vi "FSK - Listener.vi"(8 "error in (no error)":errorcluster, 11 "Queues":T1) -> (0 "error out":errorcluster)   [LabVIEW 2013]
uses:
  <vilib>/sound2/lvsound2.llb/Sound Input Task ID.ctl
  <vilib>/sound2/lvsound2.llb/Sound Data Format.ctl
  Object/FSK_OBJ - PROP.ctl
  STYPS/HDR - Queues.ctl
  <vilib>/sound2/lvsound2.llb/Sampling Mode.ctl
  <vilib>/sound2/lvsound2.llb/Sound Input Read (DBL).vi
  <vilib>/Analysis/NI_AALPro.lvlib
panel:
  out "DATA str":string
  out "DATA":string
  out "FSK":T2={"rate (bit/s)"=128.0, "bp (Bit Period)"=1e-06, "f1%"=80.0, "f2%"=20.0, "f1 (1 Freq)"=0.0, "f2 (0 Freq)"=0.0, "t (Time arry)"=[], "y1 (f1 cos arry)"=[], "y2 (f2 cos arry)"=[], "data length (B)"=0, "data size"=0, "sample size"=0.0} {"f2%" format="%#_6f"; "f1%" format="%#_6f"; "sample size" format="%#_13g"; "y2 (f2 cos arry)" format="%#_6f"; "y1 (f1 cos arry)" format="%#_6f"; "t (Time arry)" format="%#_6f"; "f2 (0 Freq)" format="%#_6f"; "f1 (1 Freq)" format="%#_6f"; "bp (Bit Period)" format="%#_13f"; "rate (bit/s)" format="%#_13g"}
  in  "PROPERTIES":T5={"device ID"=0, "number of samples/ch"=2500, "task ID"=0, "sound format"={"sample rate (S/s)"=44100.0, "number of channels"=1, "bits per sample"=16}, "DATA"=[]} {"task ID" format="%.0x"}
  out "i":i32
  out "Waveform":waveform(dbl)[](graph)
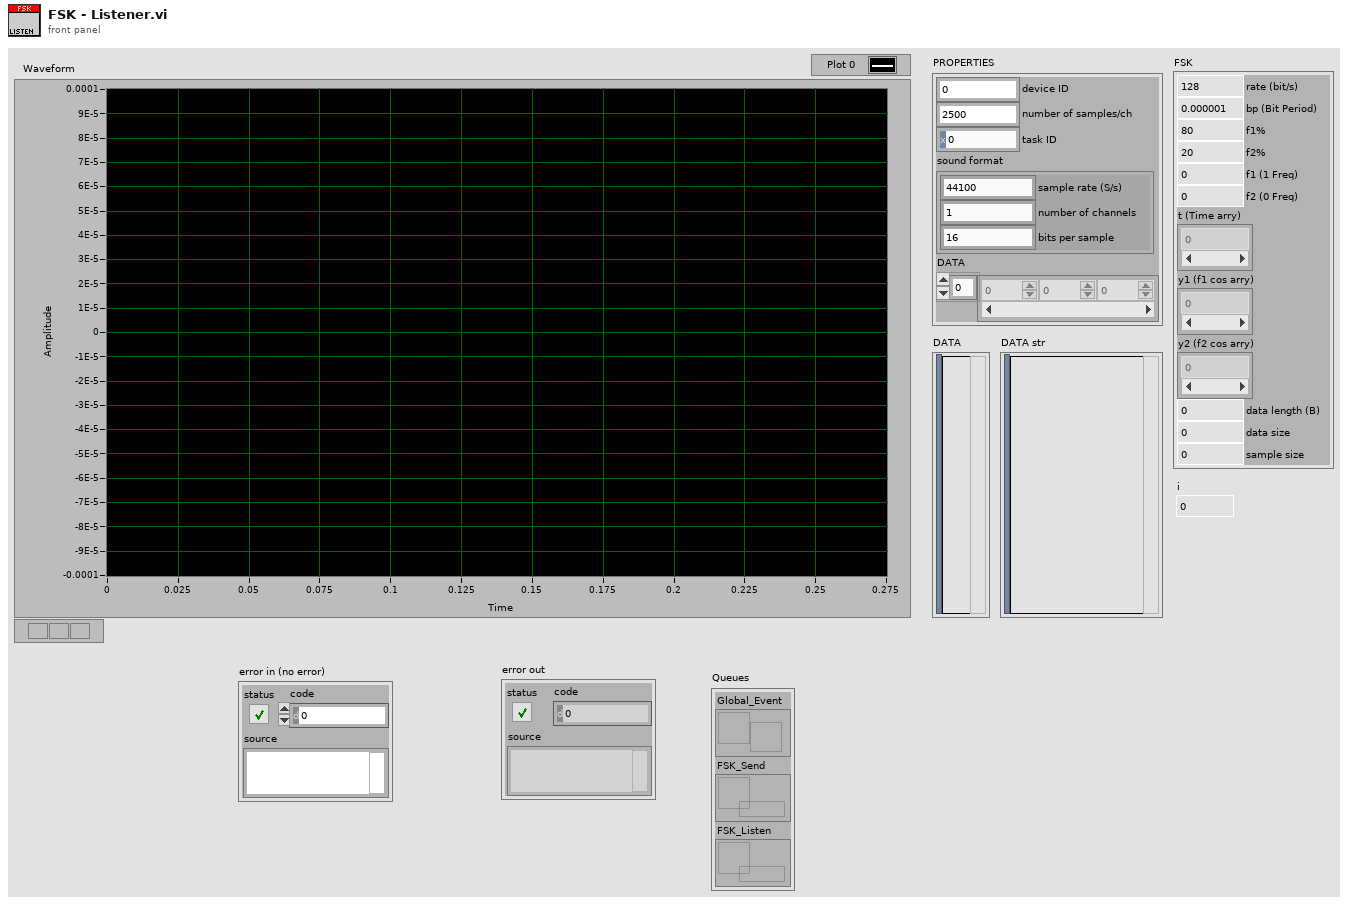
[diagram p1: front panel]
types:
  T1 = typedef "HDR - Queues.ctl" = cluster{"Global_Event":refnum<user-event>, "FSK_Send":refnum<queue>, "FSK_Listen":refnum<queue>}
  T2 = typedef "FSK_OBJ - PROP.ctl" = cluster{"rate (bit/s)":dbl, "bp (Bit Period)":dbl, "f1%":dbl, "f2%":dbl, "f1 (1 Freq)":dbl, "f2 (0 Freq)":dbl, "t (Time arry)":dbl[], "y1 (f1 cos arry)":dbl[], "y2 (f2 cos arry)":dbl[], "data length (B)":i32, "data size":i32, "sample size":dbl}
  T3 = typedef "Sound Input Task ID.ctl" = u32
  T4 = typedef "Sound Data Format.ctl" = cluster{"sample rate (S/s)":dbl, "number of channels":i32, "bits per sample":i32}
  T5 = cluster{"device ID":u32, "number of samples/ch":i32, "task ID":T3, "sound format":T4, "DATA":dbl[]}
  T6 = typedef "Sampling Mode.ctl" = i32
  T7 = typedef "AudioConfig_OBJ - PROP.ctl" = cluster{"Speaker Device ID":u32, "Microphone Device ID":u32, "sound format":T4, "number of samples/ch":i32}
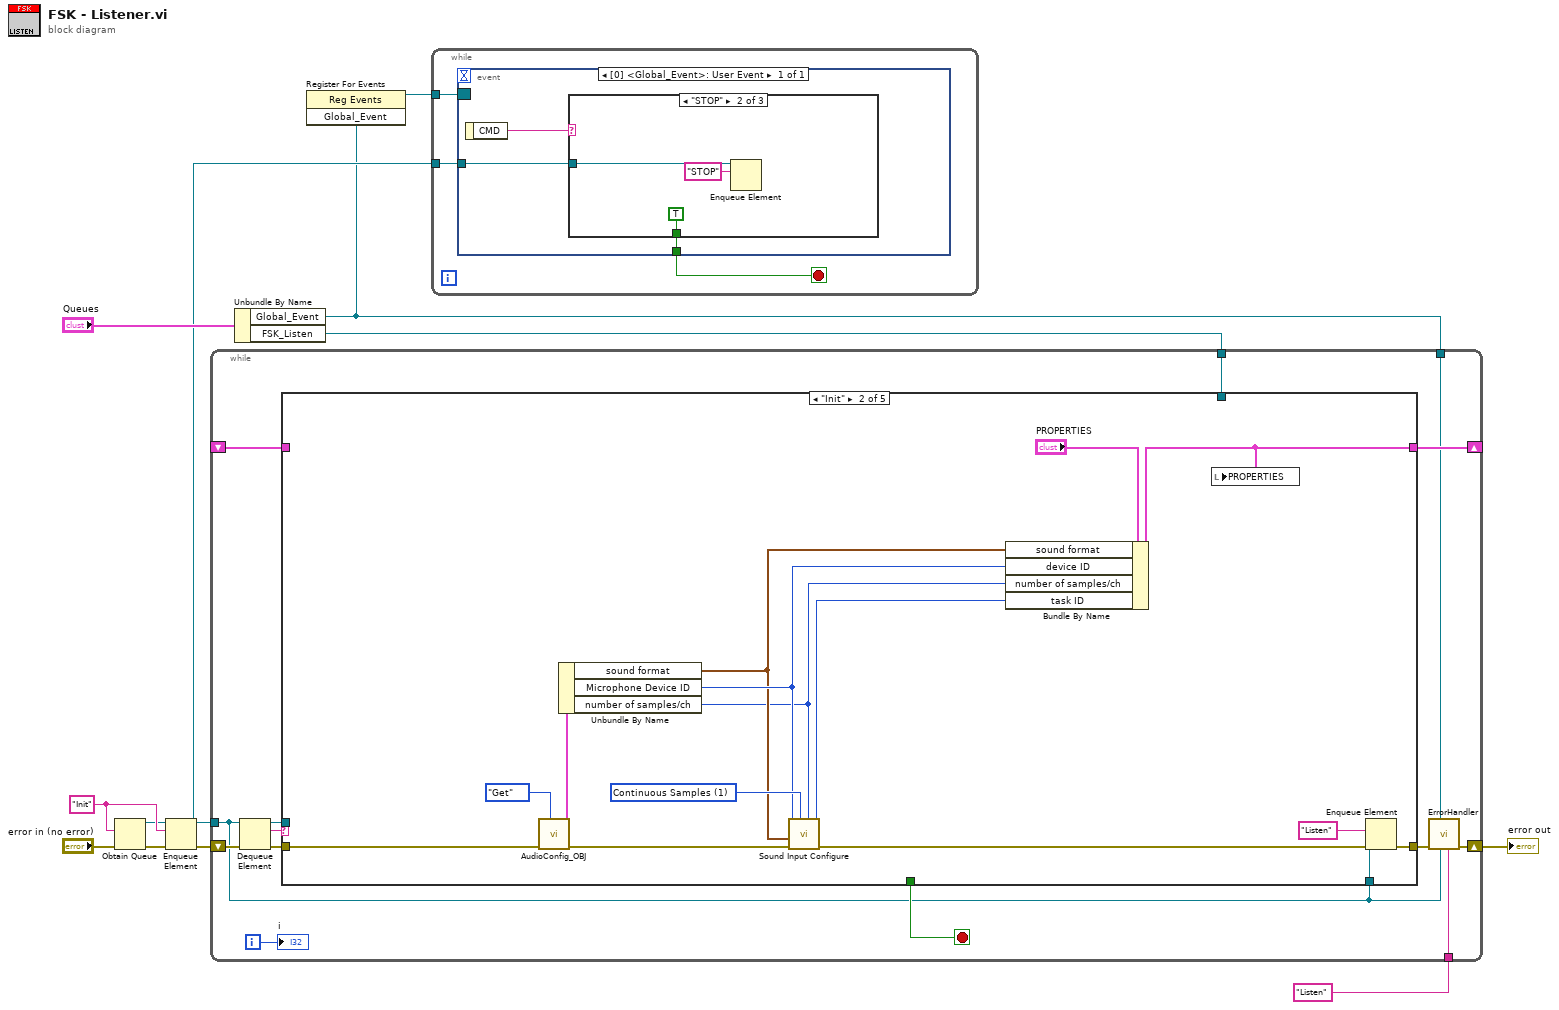
[diagram p0: block diagram]
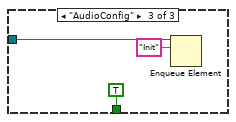
[diagram p3: hidden frame]
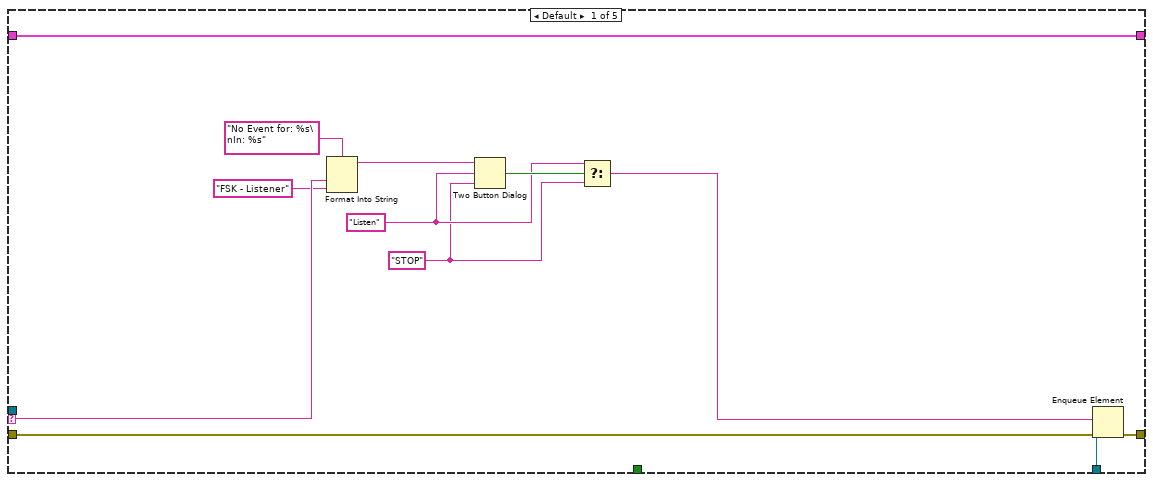
[diagram p4: hidden frame]
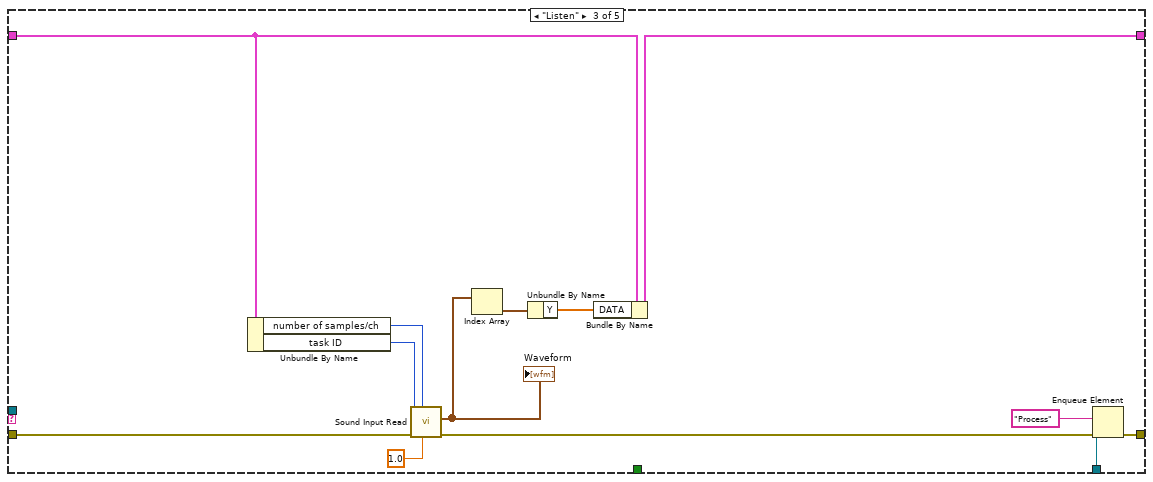
[diagram p5: hidden frame]
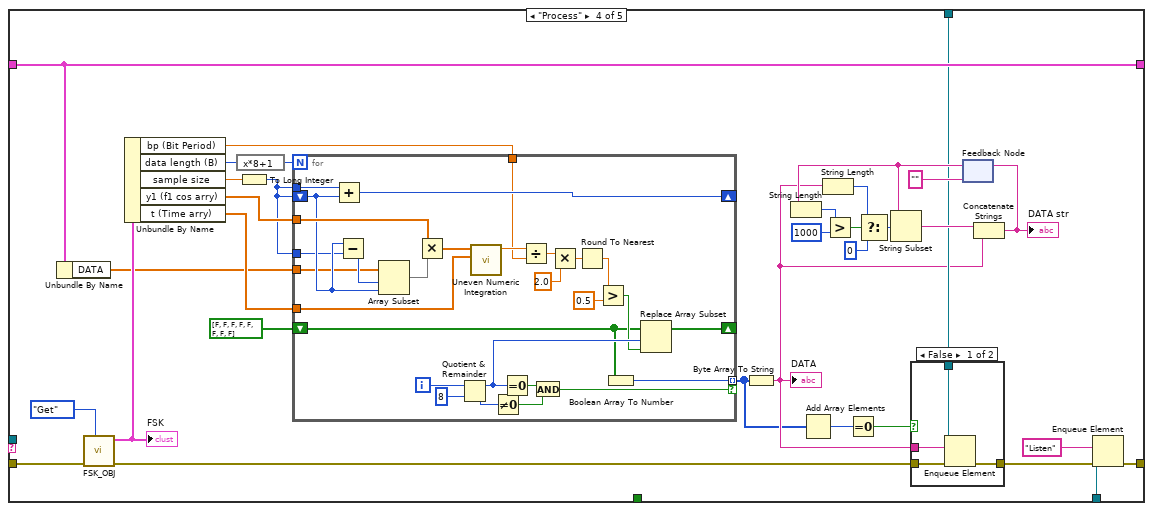
[diagram p6: hidden frame]
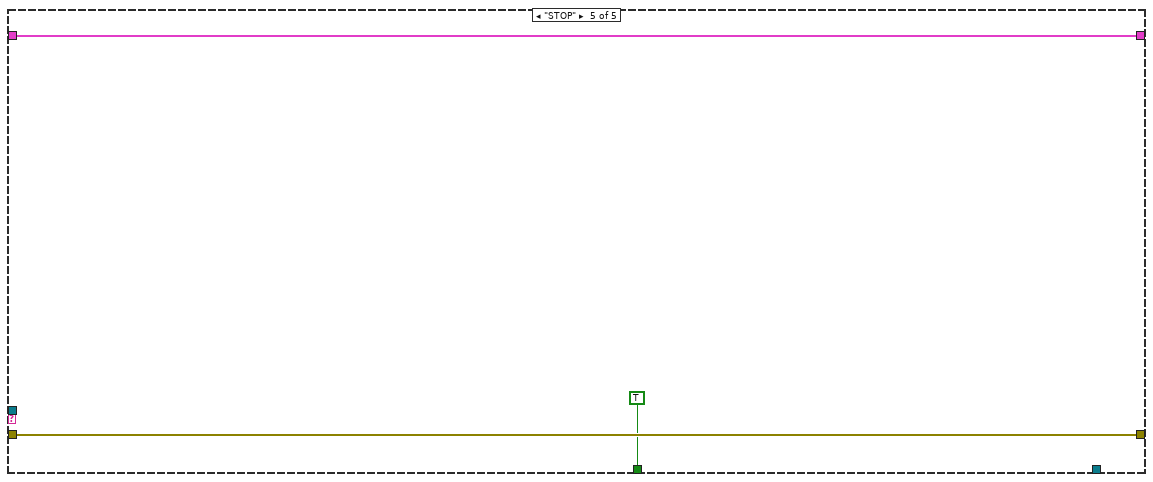
[diagram p8: hidden frame]
diagram:
  w5 = "Init"
  n1 = Obtain Queue(element data type=w5, error in (no error)="error in (no error)") -> (queue out=w4:refnum<queue>, error out=w7:errorcluster)  [unwired: 3 in, 1 out]
  n2 = Enqueue Element(queue=w4, element=w5, error in (no error)=w7) -> (queue out=w3:refnum<queue>, error out=w6:errorcluster)  [unwired: 1 in, 1 out]
  n3 = Unbundle By Name("Queues") -> ("Global_Event"=w2:refnum<user-event>, "FSK_Listen"=w9:refnum<queue>)
  n4 = while {
    shift-right: [w17] -> w12
    shift-left: w6 -> [w22]
    shift-right: [w25] -> _
    shift-left: _ -> [w24]
    tunnel: w9 -> [w23]
    tunnel: w3 -> [w14]
    tunnel: w2 -> [w15]
    tunnel: "Listen" -> [w13]
    i -> [w26]
    stop <- w18 stop-if-true
    n5 = Dequeue Element(queue=w14, error in (no error)=w22) -> (queue out=w20:refnum<queue>, element=w19:string, error out=w21:errorcluster)  [unwired: 1 in, 1 out]
    n6 = case shown="\"Init\"" w19 {
      selector: w19 -> [w37 _ _ _ _]
      tunnel: w21 -> [w29 w49 w66 w98 w134]
      tunnel: [w28 w41 w56 w70 w134] -> w16
      tunnel: [w38 w39 w60 w87 w135] -> w25
      tunnel: w24 -> [w38 _ w64 w87 w135]
      tunnel: w23 -> [_ _ _ w75 _]
      tunnel: w20 -> [_ _ _ _ _]
      tunnel: w14 -> [w30 w43 w55 w68 _]
      tunnel: [_ _ _ _ TRUE] -> w18
      frame Default {
        w32 = "Listen" ("F button name (\"Cancel\")")
        w31 = "STOP" ("F button name (\"Cancel\")")
        n7 = Format Into String(format string="No Event for: %s\nIn: %s", w37, "FSK - Listener" ("input 2")) -> (resulting string=w34:string)  [unwired: 2 in, 1 out]
        n8 = Two Button Dialog(message=w34, 1:w31, 2:w32) -> (T button?=w33:bool)
        n9 = Select(t=w32, s=w33, f=w31) -> (s? t:f=w27:string)
        n10 = Enqueue Element(queue=w30, element=w27, error in (no error)=w29) -> (error out=w28:errorcluster)  [unwired: 1 in, 2 out]
      }
      frame "Init" {
        w53 = T6 1 items=["Finite Samples", "Continuous Samples"] ("sample mode")
        n11 = call "AudioConfig_OBJ.vi"("Mode"=enum16{"Get", "Set"}."Get", "error in"=w49) -> ("error out"=w48:errorcluster, "PROPERTIES OUT"=w47:T7)  [unwired: 8 in]
        n12 = Unbundle By Name(w47) -> ("sound format"=w45:T4, "Microphone Device ID"=w46:u32, "number of samples/ch"=w44:i32)
        n13 = call <vilib>:"Sound Input Configure.vi"("number of samples/ch"=w44, "sample mode"=w53, "error in (no error)"=w48, "sound format"=w45, "device ID"=w46) -> ("error out"=w42:errorcluster, "task ID"=w51:T3)  [unwired: 5 in]
        n14 = Bundle By Name(cluster="PROPERTIES", "sound format"=w45, "device ID"=w46, "number of samples/ch"=w44, "task ID"=w51) -> (w39:T5)
        n15 = local write "PROPERTIES"(w39) -> ()
        n16 = Enqueue Element(queue=w43, element="Listen", error in (no error)=w42) -> (error out=w41:errorcluster)  [unwired: 1 in, 2 out]
      }
      frame "Listen" {
        n17 = Unbundle By Name(w64) -> ("number of samples/ch"=w59:i32, "task ID"=w63:T3)
        n18 = call-poly <vilib>:"Sound Input Read.vi"("timeout (sec)"=1.0, "number of samples/ch"=w59, "error in (no error)"=w66, "task ID"=w63) -> ("error out"=w57:errorcluster, "data"=w62:waveform(dbl)[])  [unwired: 5 in, 1 out]
        "Waveform" <- w62
        n19 = Index Array(array=w62) -> (element=w61:waveform(dbl))  [unwired: 1 in]
        n20 = Unbundle By Name(w61) -> ("Y"=w58:dbl[])
        n21 = Bundle By Name(cluster=w64, "DATA"=w58) -> (w60:T5)
        n22 = Enqueue Element(queue=w55, element="Process", error in (no error)=w57) -> (error out=w56:errorcluster)  [unwired: 1 in, 2 out]
      }
      frame "Process" {
        n23 = Unbundle By Name(w87) -> ("DATA"=w89:dbl[])
        n24 = call "FSK_OBJ.vi"("Mode"=enum16{"Get", "Set"}."Get", "error in"=w98) -> ("error out"=w76:errorcluster, "PROPERTIES OUT"=w97:T2)  [unwired: 8 in]
        "FSK" <- w97
        n25 = Unbundle By Name(w97) -> ("bp (Bit Period)"=w93:dbl, "data length (B)"=w96:i32, "sample size"=w94:dbl, "y1 (f1 cos arry)"=w92:dbl[], "t (Time arry)"=w91:dbl[])
        n26 = expression code="x*8+1"(w96) -> (w95:i32)
        n27 = To Long Integer(number=w94) -> (32bit integer=w90:i32)
        n28 = for {
          N: w95 -> [_]
          tunnel: w92 -> [w132]
          tunnel: w89 -> [w124]
          shift-right: [w130] -> _
          shift-left: w90 -> [w125]
          tunnel: w90 -> [w131]
          tunnel: w90 -> [w121]
          tunnel: w91 -> [w117]
          tunnel: w93 -> [w123]
          shift-right: [w110] -> _
          shift-left: bool[] [FALSE, FALSE, FALSE, FALSE, FALSE, FALSE, FALSE, FALSE] ("initialized array") -> [w107]
          tunnel: [w106] -> w73 mode=indexing if=w105
          i -> [w115]
          n29 = Add(x=w131, y=w125) -> (x+y=w130:i32)
          n30 = Subtract(x=w125, y=w121) -> (x-y=w129:i32)
          n31 = Array Subset(array=w124, index=w129, length=w125) -> (w128:dbl[])
          n32 = Multiply(x=w132, y=w128) -> (x*y=w118:dbl[])
          n33 = Quotient & Remainder(x=w115, y=8) -> (x-y*floor(x/y)=w109:i32, floor(x/y)=w113:i32)
          n34 = call <vilib>:"Uneven Numeric Integration.vi"("T"=w117, "X"=w118) -> ("result"=w127:dbl)  [unwired: 8 in, 1 out]
          n35 = Not Equal To 0?(x=w113) -> (x != 0?=w111:bool)
          n36 = Equal To 0?(x=w109) -> (x = 0?=w112:bool)
          n37 = Divide(x=w127, y=w123) -> (x/y=w126:dbl)
          n38 = And(x=w112, y=w111) -> (x .and. y?=w105:bool)
          n39 = Multiply(x=w126, y=2.0) -> (x*y=w122:dbl)
          n40 = Round To Nearest(number=w122) -> (nearest integer value=w120:dbl)
          n41 = Greater?(x=w120, y=0.5) -> (0:w108:bool)
          n42 = Boolean Array To Number(Boolean array=w107) -> (number=w106:u8)
          n43 = Replace Array Subset(array=w107, new element=w108, index=w109) -> (w110:bool[])
        }
        n44 = Byte Array To String(unsigned byte array=w73) -> (string=w74:string)
        "DATA" <- w74
        n45 = Add Array Elements(numeric array=w73) -> (sum=w72:u8)
        n46 = String Length(string=w74) -> (length=w82:i32)
        n47 = Equal To 0?(x=w72) -> (x = 0?=w71:bool)
        n48 = case shown="False" w71 {
          tunnel: w76 -> [w103 w104]
          tunnel: [w102 w104] -> w69
          tunnel: w75 -> [w101 _]
          tunnel: w74 -> [w100 _]
          frame False {
            n49 = Enqueue Element(queue=w101, element=w100, error in (no error)=w103) -> (error out=w102:errorcluster)  [unwired: 1 in, 2 out]
          }
          frame True {
          }
        }
        n50 = feedback #1("" ("*(type *) &x")) -> (w78:string)
        n51 = String Length(string=w78) -> (length=w86:i32)
        n52 = Greater?(x=w86, y=1000) -> (0:w84:bool)
        n53 = Select(t=w82, s=w84, f=0) -> (s? t:f=w80:i32)
        n54 = String Subset(string=w78, offset (0)=w80) -> (substring=w79:string)  [unwired: 1 in]
        n55 = Concatenate Strings(w79, w74) -> (w77:string)
        "DATA str" <- w77
        n56 = feedback-in #1(w77) -> ()
        n57 = Enqueue Element(queue=w68, element="Listen", error in (no error)=w69) -> (error out=w70:errorcluster)  [unwired: 1 in, 2 out]
      }
      frame "STOP" {
      }
    }
    n58 = call "ErrorHandler.vi"(4:"Local Event"=w13, 6:"Local Event"=w14, "Global_Event"=w15, "error in"=w16) -> ("error out"=w17:errorcluster)  [unwired: 7 in]
    "i" <- w26
  }
  "error out" <- w12
  n59 = register-events(w2) -> (reference out=w10:refnum<event-registration>)  [unwired: 2 in, 1 out]
  n60 = while {
    tunnel: w10 -> [w138]
    tunnel: w3 -> [w136]
    stop <- w137 stop-if-true
    n61 = event shown="[0] <Global_Event>: User Event" {
      selector: w138 -> [_]
      dyn-events: _ -> [_]
      timeout: _ -> [_]
      tunnel: [w140] -> w137
      tunnel: w136 -> [w139]
      event User Event {
        n62 = event-data() -> ("CMD"=w141:string)  [unwired: 1 in]
        n63 = case shown="\"STOP\"" w141 {
          tunnel: [_ TRUE TRUE] -> w140
          tunnel: w139 -> [_ w143 w146]
          frame Default {
          }
          frame "STOP" {
            n64 = Enqueue Element(queue=w143, element="STOP") -> ()  [unwired: 2 in, 3 out]
          }
          frame "AudioConfig" {
            n65 = Enqueue Element(queue=w146, element="Init") -> ()  [unwired: 2 in, 3 out]
          }
        }
      }
    }
  }
